vi "Read Write License Request Form.vi"(0 "License Form":T1, 5 "Info File Path":path, 11 "Error in (no error)":errorcluster, 13 "Operation":enum16{"Write", "Read"}(ring)=enum."Read") -> (4 "License Form Out":T1, 6 "Info File Path":path, 15 "Error out":errorcluster)   [LabVIEW 2022 SP3]
uses:
  Controls/License Request Form.ctl
  <vilib>/Utility/sysdir.llb/System Directory Type.ctl
panel:
  out "ROT'd string":string
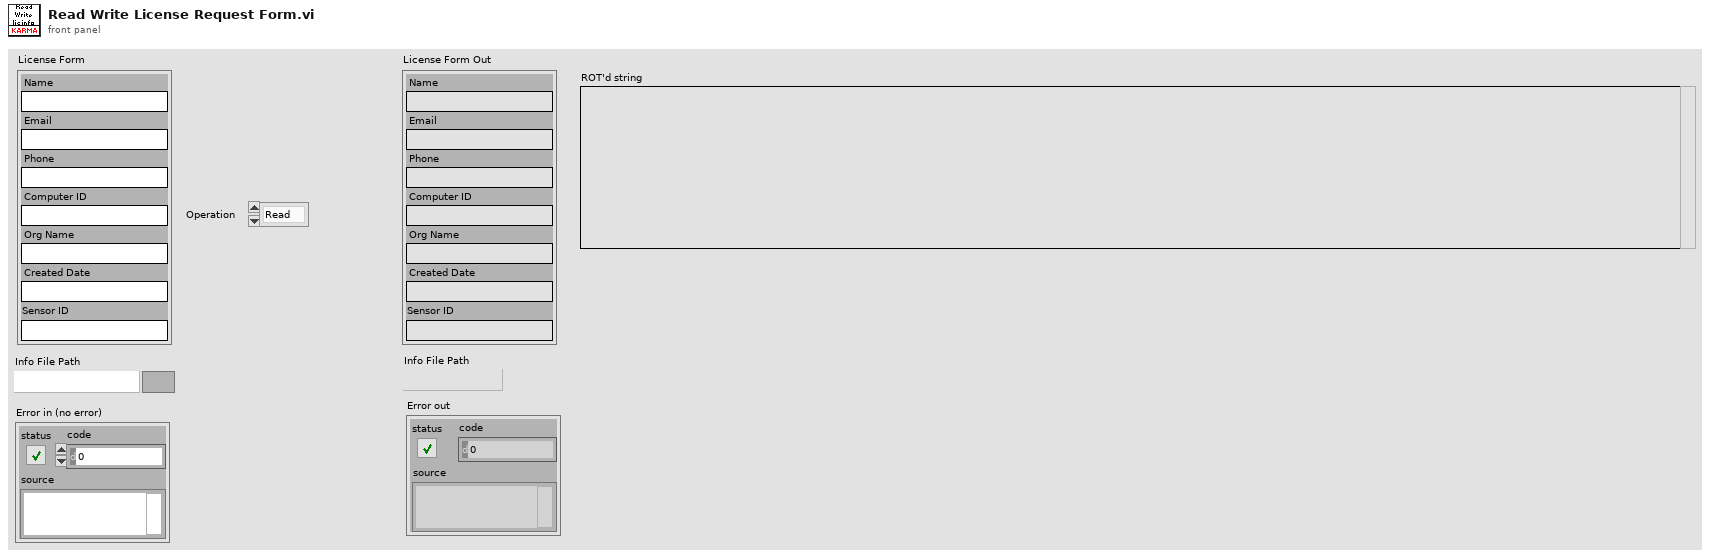
[diagram p1: front panel]
types:
  T1 = typedef "License Request Form.ctl" = cluster{"Name":string, "Email":string, "Phone":string, "Computer ID":string, "Org Name":string, "Created Date":string, "Sensor ID":string}
  T2 = enum16{"open", "replace", "create", "open or create", "replace or create", "replace or create with confirmation"}
  T3 = typedef "System Directory Type.ctl" = i32
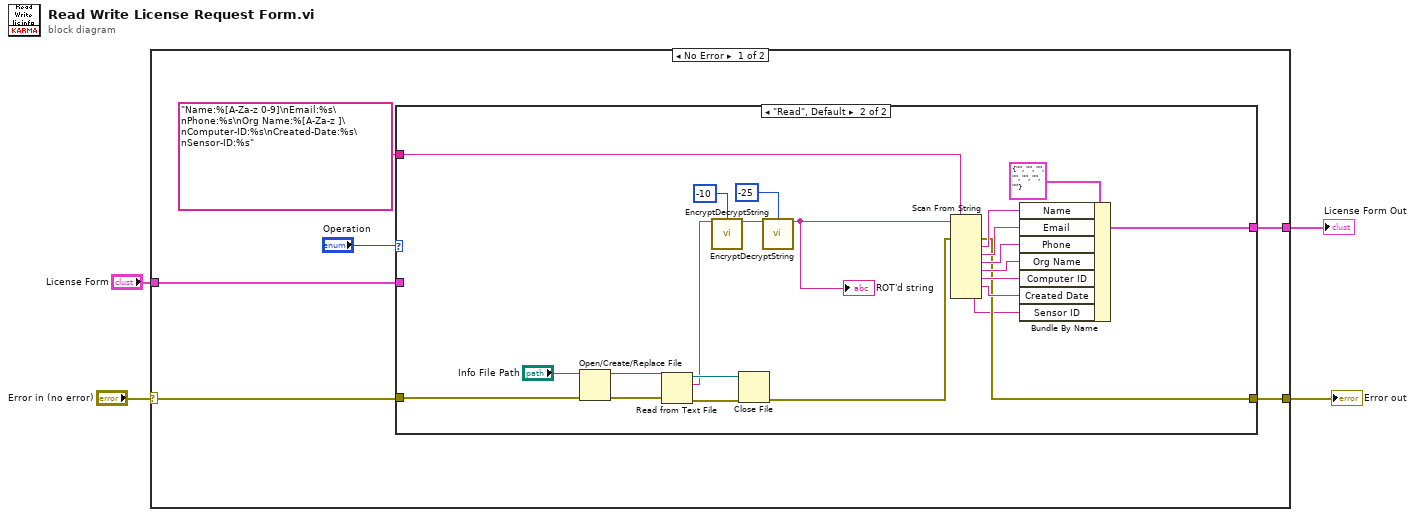
[diagram p0: block diagram]
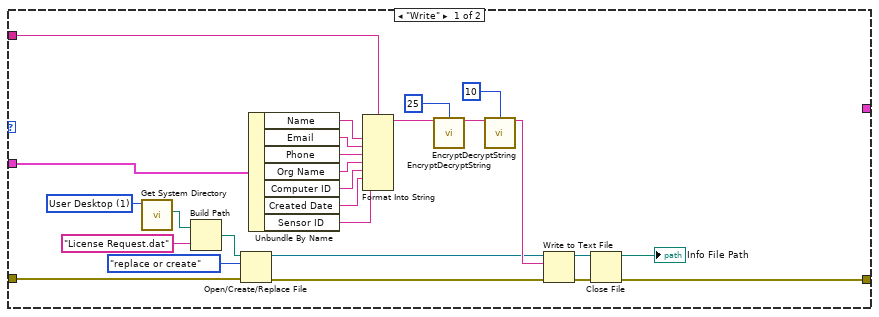
[diagram p2: hidden frame]
diagram:
  n1 = case shown="No Error" "Error in (no error)" {
    selector: "Error in (no error)" -> [w7 w60]
    tunnel: [w8 w60] -> w4
    tunnel: "License Form" -> [w10 _]
    tunnel: [w5 _] -> w1
    frame No Error {
      n2 = case shown="\"Read\", Default" "Operation" {
        tunnel: w10 -> [w36 _]
        tunnel: [w15 w40] -> w8
        tunnel: w7 -> [w22 w55]
        tunnel: "Name:%[A-Za-z 0-9]\nEmail:%s\nPhone:%s\nOrg Name:%[A-Za-z ]\nComputer-ID:%s\nCreated-Date:%s\nSensor-ID:%s" ("format string") -> [w13 w54]
        tunnel: [_ w43] -> w5
        frame "Write" {
          w19 = T3 1 items=["User Home"=0, "User Desktop"=1, "User Documents"=2, "User Application Data"=3, "User Preferences"=4, "User Temporary"=5, "Public Documents"=6, "Public Application Data"=7, "Public Preferences"=8, "Public Cache"=13, "System Core Libraries"=9, "System Installed Libraries"=10, "Application Files"=11, "Boot Volume Root"=12] ("system directory type")
          n3 = call <vilib>:"Get System Directory.vi"("system directory type"=w19) -> ("system directory"=w23:path)  [unwired: 10 in]
          n4 = Build Path(base path=w23, name or relative path="License Request.dat") -> (appended path=w24:path)
          n5 = Open/Create/Replace File(file path (use dialog)=w24, error in=w22, operation (0:open)=T2."replace or create") -> (refnum out=w17:refnum<file>, error out=w18:errorcluster)  [unwired: 3 in, 1 out]
          n6 = Unbundle By Name(w36) -> ("Name"=w35:string, "Email"=w34:string, "Phone"=w33:string, "Org Name"=w32:string, "Computer ID"=w31:string, "Created Date"=w30:string, "Sensor ID"=w11:string)
          n7 = Format Into String(format string=w13, w35, w34, w33, w32, w31, w30, w11) -> (resulting string=w29:string)  [unwired: 2 in, 1 out]
          n8 = call "EncryptDecryptString.vi"("Original"=w29, "ROT by..."=25) -> ("ROT'd string"=w27:string)  [unwired: 13 in]
          n9 = call "EncryptDecryptString.vi"("Original"=w27, "ROT by..."=10) -> ("ROT'd string"=w25:string)  [unwired: 13 in]
          n10 = Write to Text File(file (use dialog)=w17, text=w25, error in=w18) -> (refnum out=w14:refnum<file>, error out=w16:errorcluster)  [unwired: 1 in, 1 out]
          n11 = Close File(refnum=w14, error in=w16) -> (path=→"Info File Path":path, error out=w15:errorcluster)
        }
        frame "Read", Default {
          n12 = Open/Create/Replace File(file path (use dialog)="Info File Path", error in=w55) -> (refnum out=w57:refnum<file>, error out=w59:errorcluster)  [unwired: 4 in, 1 out]
          n13 = Read from Text File(file (use dialog)=w57, error in=w59) -> (refnum out=w42:refnum<file>, text=w38:string, error out=w58:errorcluster)  [unwired: 2 in, 1 out]
          n14 = call "EncryptDecryptString.vi"("Original"=w38, "ROT by..."=-10) -> ("ROT'd string"=w51:string)  [unwired: 13 in]
          n15 = Close File(refnum=w42, error in=w58) -> (error out=w41:errorcluster)  [unwired: 1 out]
          n16 = call "EncryptDecryptString.vi"("Original"=w51, "ROT by..."=-25) -> ("ROT'd string"=w39:string)  [unwired: 13 in]
          "ROT'd string" <- w39
          n17 = Scan From String(format string=w54, input string=w39, error in=w41) -> (error out=w40:errorcluster, output 1=w49:string, output 2=w48:string, output 3=w47:string, output 4=w46:string, output 5=w45:string, output 6=w44:string, output 7=w37:string)  [unwired: 8 in, 2 out]
          n18 = Bundle By Name(cluster=T1 {"Name"="", "Email"="", "Phone"="", "Computer ID"="", "Org Name"="", "Created Date"="", "Sensor ID"=""} ("License Form 2"), "Name"=w49, "Email"=w48, "Phone"=w47, "Org Name"=w46, "Computer ID"=w45, "Created Date"=w44, "Sensor ID"=w37) -> (w43:T1)
        }
      }
    }
    frame Error {
    }
  }
  "Error out" <- w4
  "License Form Out" <- w1
